vi "Check if Feed is Registered.vi"(8 "error in":errorcluster, 11 "feed URI":string) -> (0 "error out":errorcluster, 2 "feed URI registered?":bool, 3 "feed URI out":string)   [LabVIEW 2014, in "NIPM_API.lvlib"]
uses:
  NIPM_API.lvlib
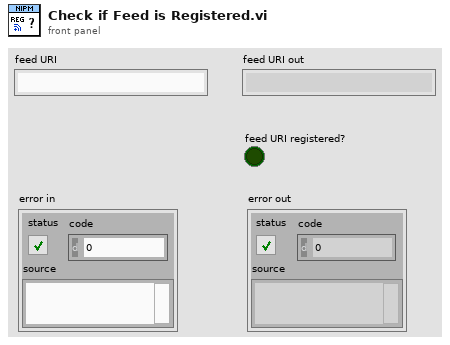
[diagram p1: front panel]
types:
  T1 = typedef "NIPM_API.lvlib/feed.ctl" = cluster{"Name":string, "URI":string}
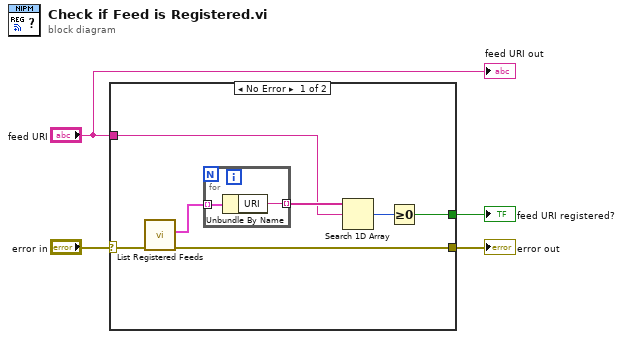
[diagram p0: block diagram]
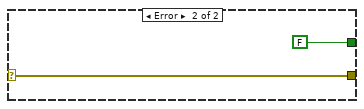
[diagram p2: hidden frame]
diagram:
  n1 = case shown="No Error" "error in" {
    selector: "error in" -> [w11 w15]
    tunnel: [w10 w15] -> w3
    tunnel: "feed URI" -> [w7 _]
    tunnel: [w5 FALSE] -> w1
    frame No Error {
      n2 = call "List Registered Feeds.vi"("error in"=w11) -> ("error out"=w10:errorcluster, "registered feeds"=w9:T1[])  [unwired: 9 in]
      n3 = for {
        tunnel: w9 -> [w13] mode=indexing
        tunnel: [w12] -> w8 mode=indexing
        n4 = Unbundle By Name(w13) -> ("URI"=w12:string)
      }
      n5 = Search 1D Array(1D array=w8, element=w7) -> (index of element=w6:i32)  [unwired: 1 in]
      n6 = Greater Or Equal To 0?(x=w6) -> (x >= 0?=w5:bool)
    }
    frame Error {
    }
  }
  "error out" <- w3
  "feed URI registered?" <- w1
  "feed URI out" <- "feed URI"
